vi "WTSensorChecker.vi"() -> ()   [LabVIEW 2017]
panel:
  in  "Sampling Frequency (Hz)":sgl=5000.0
  in  "Record_Data":bool caption="Record Data:"
  out "ElapsedTime":string caption="Elapsed Time:"
  out "StratTime":string caption="Strat Time:"
  out "LATD":cluster{"Double":dbl, "Double":dbl}(graph) caption="Lab Atmospheric Density"
  out "LATT":cluster{"Double":dbl, "Double":dbl}(graph) caption="Lab Atmospheric Temperature"
  out "LATP":cluster{"Double":dbl, "Double":dbl}(graph) caption="Lab Atmospheric Pressure"
  in  "Stop":bool caption="Log Data:"
  # "Wind Tunnel Sensor Data Viewer"
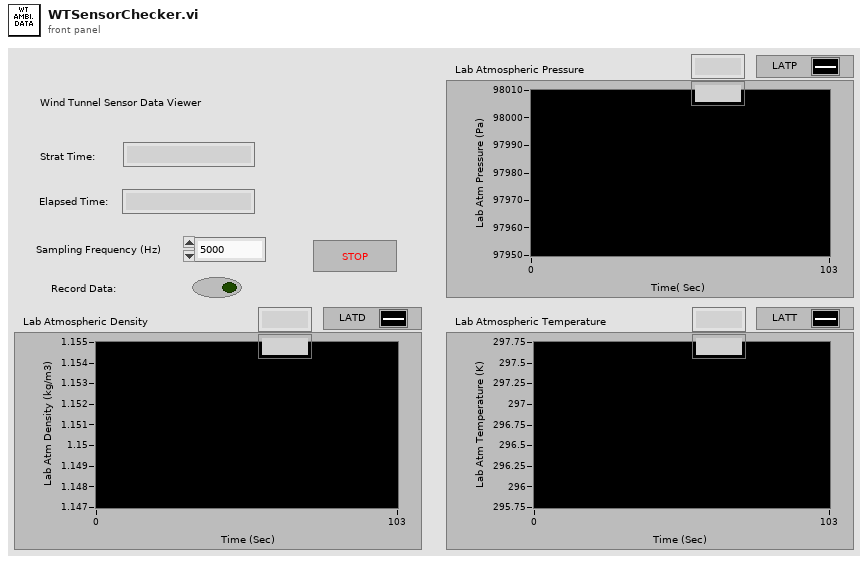
[diagram p1: front panel]
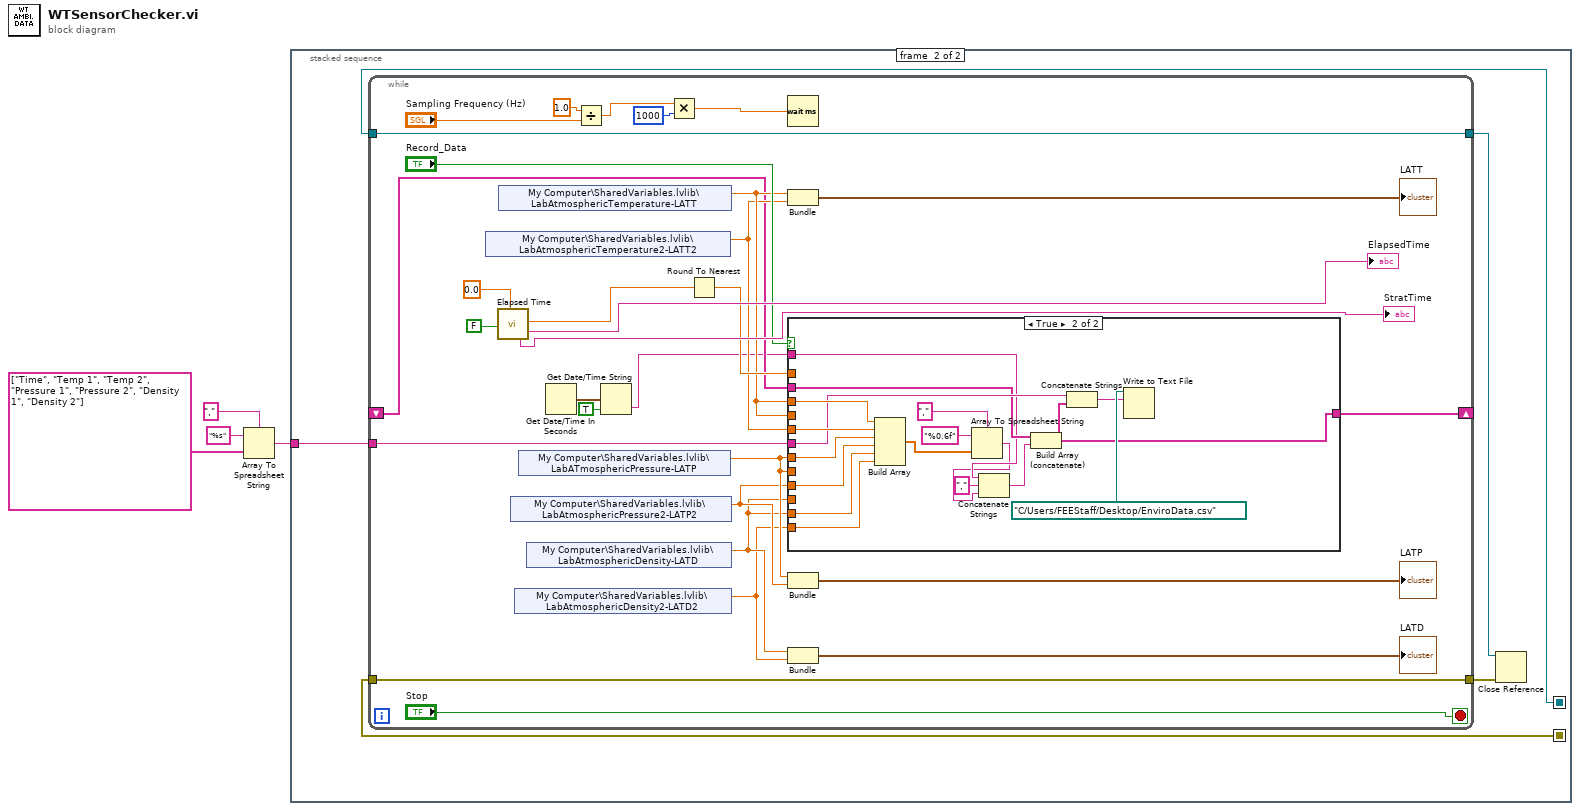
[diagram p0: block diagram]
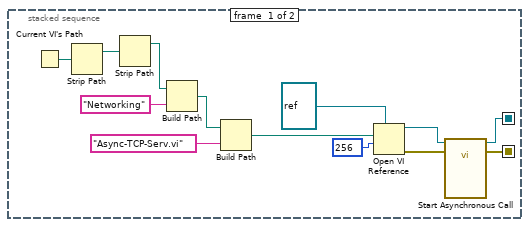
[diagram p2: hidden frame]
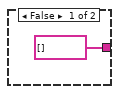
[diagram p3: hidden frame]
diagram:
  n1 = Array To Spreadsheet String(delimiter (Tab)=",", array=string[] ["Time", "Temp 1", "Temp 2", "Pressure 1", "Pressure 2", "Density 1", "Density 2"], 3:"%s" ("delimiter (Tab)")) -> (spreadsheet string=w4:string)
  n2 = stacked-sequence {
    seq-local: [w11 _] -> [_ w22]
    seq-local: [w10 _] -> [_ w21]
    tunnel: w4 -> [_ w18]
    frame #0 {
      n3 = Current VI's Path() -> (path=w9:path)
      n4 = Strip Path(path=w9) -> (stripped path=w8:path)  [unwired: 1 out]
      n5 = Strip Path(path=w8) -> (stripped path=w7:path)  [unwired: 1 out]
      n6 = Build Path(base path=w7, name or relative path="Networking") -> (appended path=w5:path)
      n7 = Build Path(base path=w5, name or relative path="Async-TCP-Serv.vi") -> (appended path=w16:path)
      n8 = Open VI Reference(type specifier VI Refnum (for type only)=refnum<vi> refnum, vi path=w16, options=256) -> (vi reference=w13:refnum<vi>, error out=w12:errorcluster)  [unwired: 3 in]
      n9 = call-by-ref "Start Asynchronous Call"(reference=w13, error in=w12) -> (reference out=w11:refnum<vi>, error out=w10:errorcluster)  [unwired: 12 in]
    }
    frame #1 {
      n10 = while {
        tunnel: w22 -> [w40]
        tunnel: w21 -> [w39]
        tunnel: [w40] -> w20
        tunnel: [w39] -> w19
        tunnel: w18 -> [w28]
        shift-right: [w27] -> _
        shift-left: _ -> [w26]
        stop <- "Stop" stop-if-true
        n11 = shared-variable "My Computer\\SharedVariables.lvlib\\LabAtmosphericTemperature2-LATT2"() -> (w33:dbl)  [unwired: 1 in, 1 out]
        n12 = call "Elapsed Time"("Auto Reset"=FALSE, "Set Start Time (s)"=0.0) -> ("Start Time Text"=→"StratTime":string, "Elapsed Time (s)"=w52:dbl, "Elapsed Time Text"=→"ElapsedTime":string)  [unwired: 10 in, 5 out]
        n13 = shared-variable "My Computer\\SharedVariables.lvlib\\LabAtmosphericTemperature-LATT"() -> (w34:dbl)  [unwired: 1 in, 1 out]
        n14 = shared-variable "My Computer\\SharedVariables.lvlib\\LabAtmosphericPressure2-LATP2"() -> (w31:dbl)  [unwired: 1 in, 1 out]
        n15 = shared-variable "My Computer\\SharedVariables.lvlib\\LabAtmosphericDensity2-LATD2"() -> (w29:dbl)  [unwired: 1 in, 1 out]
        n16 = shared-variable "My Computer\\SharedVariables.lvlib\\LabATmosphericPressure-LATP"() -> (w32:dbl)  [unwired: 1 in, 1 out]
        n17 = shared-variable "My Computer\\SharedVariables.lvlib\\LabAtmosphericDensity-LATD"() -> (w30:dbl)  [unwired: 1 in, 1 out]
        n18 = Get Date/Time In Seconds() -> (seconds since 1Jan1904=w25:timestamp)
        n19 = Divide(x=sgl 1.0, y="Sampling Frequency (Hz)") -> (x/y=w41:sgl)
        n20 = Get Date/Time String(seconds (now)=w25, want seconds? (F)=TRUE) -> (time string=w23:string)  [unwired: 1 in, 1 out]
        n21 = Multiply(x=w41, y=u32 1000) -> (x*y=w44:sgl)
        n22 = Round To Nearest(number=w52) -> (nearest integer value=w38:dbl)
        n23 = Wait (ms)(milliseconds to wait=w44) -> ()  [unwired: 1 out]
        n24 = Bundle("Double"=w34, "Double"=w33) -> (→"LATT":cluster{"Double":dbl, "Double":dbl})  [unwired: 1 in]
        n25 = case shown="True" "Record_Data" {
          tunnel: w38 -> [_ _]
          tunnel: w34 -> [_ _]
          tunnel: w32 -> [_ _]
          tunnel: w30 -> [_ _]
          tunnel: w34 -> [_ w71]
          tunnel: w33 -> [_ w70]
          tunnel: w32 -> [_ w69]
          tunnel: w31 -> [_ w68]
          tunnel: w30 -> [_ w67]
          tunnel: w29 -> [_ w66]
          tunnel: w28 -> [_ w61]
          tunnel: [string[] [] w58] -> w27
          tunnel: w26 -> [_ w59]
          tunnel: w23 -> [_ w57]
          frame False {
          }
          frame True {
            n26 = Build Array(w71, w70, w69, w68, w67, w66) -> (w65:dbl[])
            n27 = Array To Spreadsheet String(delimiter (Tab)=",", array=w65, 3:"%0.6f" ("format string")) -> (spreadsheet string=w55:string)
            n28 = Concatenate Strings(w57, "," ("string"), w55) -> (w54:string)
            n29 = Build Array (concatenate)(w59, w54) -> (w58:string[])
            n30 = Concatenate Strings(w61, w58) -> (w60:string)
            n31 = Write to Text File(file (use dialog)=path "C:/Users/FEEStaff/Desktop/EnviroData.csv", text=w60) -> ()  [unwired: 2 in, 3 out]
          }
        }
        n32 = Bundle("Double"=w32, "Double"=w31) -> (→"LATP":cluster{"Double":dbl, "Double":dbl})  [unwired: 1 in]
        n33 = Bundle("Double"=w30, "Double"=w29) -> (→"LATD":cluster{"Double":dbl, "Double":dbl})  [unwired: 1 in]
      }
      n34 = Close Reference(reference=w20, error in (no error)=w19) -> ()  [unwired: 1 out]
    }
  }
